vi "TR_Filter_magnets_coordinates_(offline).vi"(7 "Data filtering":T1={"Filter type"=enum."Savitzky-Golay", "Length"=41, "Order"=3} {"Order" min=3 max=11 step=2; "Length" min=5 max=301 step=2}, 8 "error in (no error)":errorcluster, 11 "Magnets raw coordinates in":dbl[][](array[numeric])) -> (0 "error out":errorcluster, 3 "Magnets filtered coordinates out":dbl[][](array[numeric]))   [LabVIEW 2018, in "Tracks Repair.lvlib"]
uses:
  Tracks Repair.lvlib
  SubVi's/Controls/CTL_Filter_selector.ctl
  <vilib>/Analysis/3filter.llb/Savitzky-Golay Filter (DBL).vi
  <vilib>/Analysis/NI_AALBase.lvlib
  Tracker.lvlib
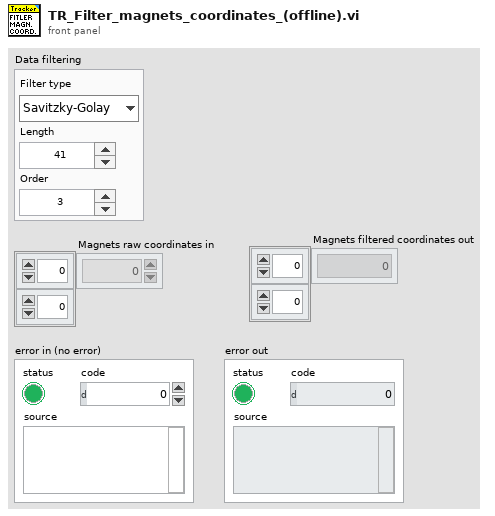
[diagram p1: front panel]
types:
  T1 = typedef "Tracker.lvlib/CTL_Filter_selector.ctl" = cluster{"Filter type":enum16{"None", "Savitzky-Golay"}, "Length":i32, "Order":i32}
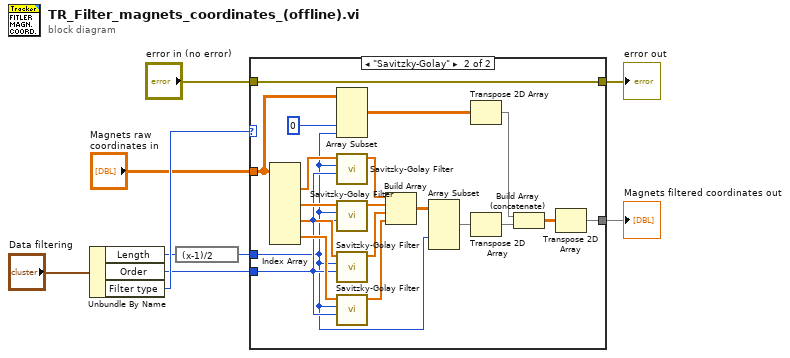
[diagram p0: block diagram]
diagram:
  n1 = Unbundle By Name("Data filtering") -> ("Length"=w4:i32, "Order"=w6:i32, "Filter type"=w7:enum16{"None", "Savitzky-Golay"})
  n2 = expression code="(x-1)/2"(w4) -> (w5:i32)
  n3 = case shown="\"Savitzky-Golay\"" w7 {
    tunnel: "Magnets raw coordinates in" -> [w11 w21]
    tunnel: w5 -> [_ w15]
    tunnel: w6 -> [_ w27]
    tunnel: [w11 w12] -> w2
    tunnel: [w10 w22] -> w8
    tunnel: "error in (no error)" -> [w10 w22]
    frame "None", Default {
    }
    frame "Savitzky-Golay" {
      n4 = Index Array(array=w21) -> (element #1=w31:dbl[], element #2=w30:dbl[], element #3=w29:dbl[], element #4=w28:dbl[])  [unwired: 8 in]
      n5 = Array Subset(array=w21, index (col)=0 ("index"), length (col)=w15) -> (w19:dbl[][])  [unwired: 2 in]
      n6 = call-poly <vilib>:"Savitzky-Golay Filter.vi"("polynomial order"=w27, "side points"=w15, "X"=w31) -> ("Filtered X"=w26:dbl[])  [unwired: 7 in, 1 out]
      n7 = call-poly <vilib>:"Savitzky-Golay Filter.vi"("polynomial order"=w27, "side points"=w15, "X"=w30) -> ("Filtered X"=w25:dbl[])  [unwired: 7 in, 1 out]
      n8 = call-poly <vilib>:"Savitzky-Golay Filter.vi"("polynomial order"=w27, "side points"=w15, "X"=w29) -> ("Filtered X"=w24:dbl[])  [unwired: 7 in, 1 out]
      n9 = call-poly <vilib>:"Savitzky-Golay Filter.vi"("polynomial order"=w27, "side points"=w15, "X"=w28) -> ("Filtered X"=w23:dbl[])  [unwired: 7 in, 1 out]
      n10 = Build Array(w26, w25, w24, w23) -> (w20:dbl[][])
      n11 = Array Subset(array=w20, index (col)=w15) -> (w18:dbl[][])  [unwired: 3 in]
      n12 = Transpose 2D Array(2D array=w19) -> (transposed array=w14:dbl[][])
      n13 = Transpose 2D Array(2D array=w18) -> (transposed array=w13:dbl[][])
      n14 = Build Array (concatenate)(w14, w13) -> (w17:dbl[][])
      n15 = Transpose 2D Array(2D array=w17) -> (transposed array=w12:dbl[][])
    }
  }
  "error out" <- w8
  "Magnets filtered coordinates out" <- w2
